vi "Get Linked Version.vi"(8 "error in":errorcluster) -> (0 "error out":errorcluster, 3 "Version":T1)   [LabVIEW 2014, in "LibSDL2_Mixer.lvlib"]
uses:
  LibSDL2_Mixer.lvlib
  LibSDL2 Wrapper/Controls/Version.ctl
  <vilib>/Utility/importsl/GetValueByPointer/datatype.ctl
  <vilib>/Utility/importsl/GetValueByPointer/GetValueByPointer.xnode
  LibSDL2 Wrapper/LibSDL2.lvlib
  LibSDL2 Wrapper/DLL/SDL2_mixer.dll
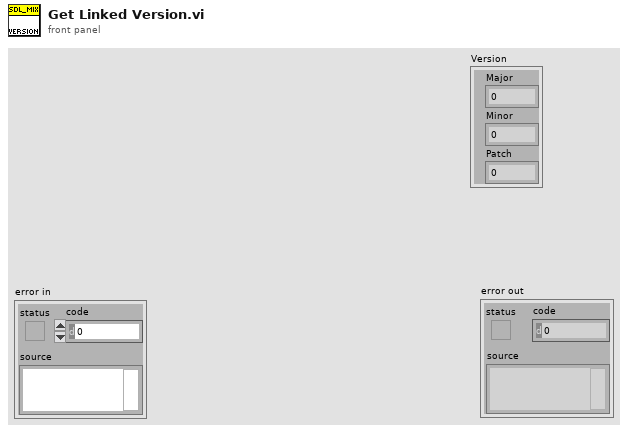
[diagram p1: front panel]
types:
  T1 = typedef "LibSDL2.lvlib/Version.ctl" = cluster{"Major":u8, "Minor":u8, "Patch":u8}
  T2 = enum32{"pack1", "pack2", "pack4", "pack8", "pack16"}
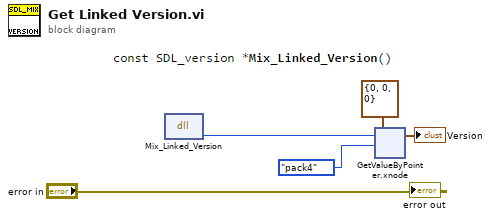
[diagram p0: block diagram]
diagram:
  n1 = dll-call lib="C:/dev/PGS/LabSDL2/Source/Libraries/LibSDL2 Wrapper/DLL/SDL2_mixer.dll" fn="Mix_Linked_Version"() -> ("return type"=w3:u32)  [unwired: 3 in, 2 out]
  n2 = xnode "GetValueByPointer.xnode"("Pointer"=w3, "InputType"=T1 {"Major"=0, "Minor"=0, "Patch"=0} ("Version"), "PackType"=T2."pack4") -> ("Output"=→"Version":T1)  [unwired: 1 in, 1 out]
  "error out" <- "error in"
